vi "LPush.vi"(0 "reference in":refnum<class "Redis.lvclass">, 1 "Key":string, 7 "Values":string[](array[string]), 11 "Error In":errorcluster) -> (4 "reference out":refnum<class "Redis.lvclass">, 8 "Return":i64, 15 "Error Out":errorcluster)   [LabVIEW 2020, in "Redis.lvclass"]
doc: "<b>LPUSH</b>\n\nInsert all the specified values at the head of the list stored at key. If key does not exist, it is created as empty list before performing the push operations. When key holds a value that is not a list, an error is returned.\n\nIt is possible to push multiple elements using a single command call just specifying multiple arguments at the end of the command. Elements are inserted one after the other to the head of the list, from the leftmost element to the rightmost element. So for instance the command LPUSH mylist a b c will result into a list containing c as first element, b as second element and a as third element."
uses:
  Redis.lvclass
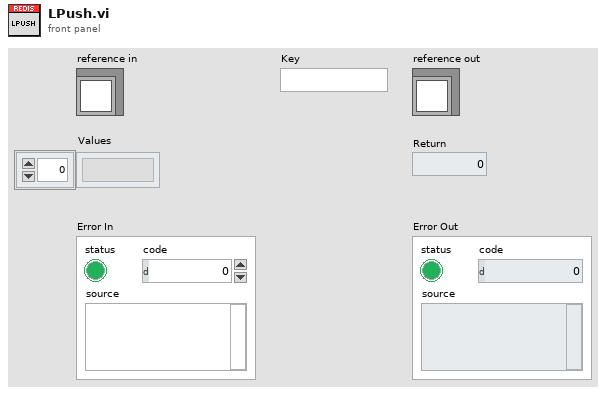
[diagram p1: front panel]
types:
  T1 = typedef "Redis.lvclass/RedisDataType.ctl" = cluster{"Reply Type":T2, "Integer":i64, "String":string, "Multibulk":variant[], "StringData":string[]}
  T2 = typedef "Redis.lvclass/ReplyDataTypeEnum.ctl" = enum16{"None", "Error", "Status", "Nil", "Integer", "String", "Multibulk"}
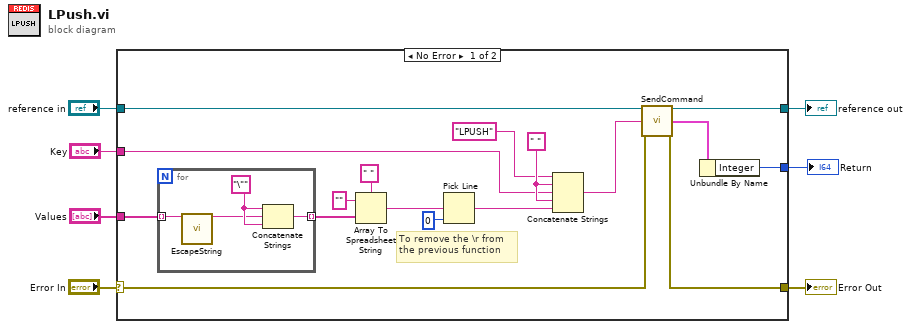
[diagram p0: block diagram]
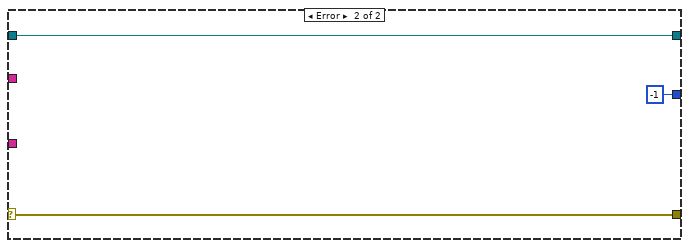
[diagram p2: hidden frame]
diagram:
  n1 = case shown="No Error" "Error In" {
    selector: "Error In" -> [w22 w31]
    tunnel: [w21 w31] -> w6
    tunnel: [w24 w30] -> w4
    tunnel: "reference in" -> [w23 w30]
    tunnel: "Key" -> [w11 _]
    tunnel: "Values" -> [w10 _]
    tunnel: [w8 i64 -1 ("Integer")] -> w1
    frame No Error {
      w14 = " "
      # "To remove the \\r from\nthe previous function"
      n2 = for {
        tunnel: w10 -> [w26] mode=indexing
        tunnel: [w28] -> w13 mode=indexing
        w27 = "\""
        n3 = call "EscapeString.vi"("String"=w26) -> ("Escaped String"=w25:string)  [unwired: 13 in, 1 out]
        n4 = Concatenate Strings(w27, w25, w27) -> (w28:string)
      }
      n5 = Array To Spreadsheet String(delimiter (Tab)=" ", array=w13, 3:"" ("format string")) -> (spreadsheet string=w16:string)
      n6 = Pick Line(multi-line string=w16, line index=0) -> (output string=w17:string)  [unwired: 1 in]
      n7 = Concatenate Strings("LPUSH", w14, w11, w14, w17) -> (w9:string)
      n8 = call "SendCommand.vi"("reference in"=w23, "Command"=w9, "Error In"=w22) -> ("reference out"=w24:refnum<class "Redis.lvclass">, "Data"=w20:T1, "Error Out"=w21:errorcluster)  [unwired: 10 in]
      n9 = Unbundle By Name(w20) -> ("Integer"=w8:i64)
    }
    frame Error {
    }
  }
  "Error Out" <- w6
  "reference out" <- w4
  "Return" <- w1
